vi "decimate.vi"(10 "Waveform":waveform(dbl), 11 "Divide by":i32=20) -> (3 "output waveform":waveform(dbl))   [LabVIEW 2014]
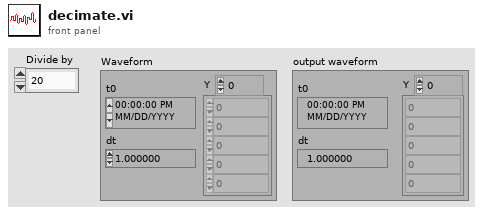
[diagram p1: front panel]
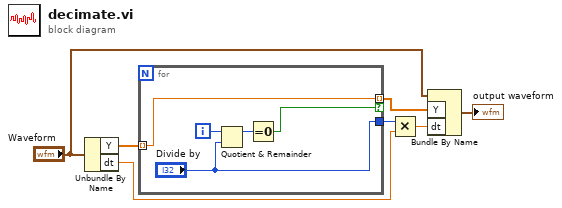
[diagram p0: block diagram]
diagram:
  n1 = Unbundle By Name("Waveform") -> ("Y"=w2:dbl[], "dt"=w4:dbl)
  n2 = for {
    tunnel: w2 -> [w8] mode=indexing
    tunnel: ["Divide by"] -> w5
    tunnel: [w8] -> w7 mode=indexing if=w9
    i -> [w11]
    n3 = Quotient & Remainder(x=w11, y="Divide by") -> (x-y*floor(x/y)=w12:i32)  [unwired: 1 out]
    n4 = Equal To 0?(x=w12) -> (x = 0?=w9:bool)
  }
  n5 = Multiply(x=w5, y=w4) -> (x*y=w3:dbl)
  n6 = Bundle By Name(cluster="Waveform", "Y"=w7, "dt"=w3) -> (→"output waveform":waveform(dbl))
